vi "44xxRefClk.vi"(8 "error in (no error)":errorcluster, 9 "DAQ Type":T1, 10 "ActiveDev":tag, 11 "Refnum in":refnum<k21>) -> (0 "error out":errorcluster, 2 "RefClk.Src":tag, 3 "Refnum out":refnum<k21>)   [LabVIEW 2016, in "Instrument.Lockin.lvclass"]
uses:
  Instrument.Lockin.lvclass
  Typedefs/DAQType-enum.ctl
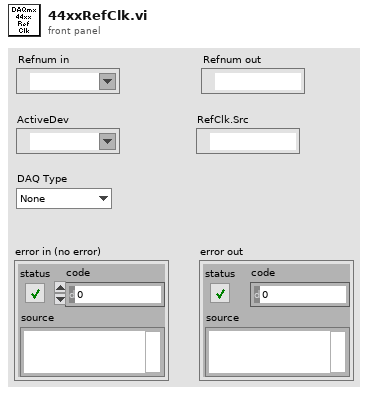
[diagram p1: front panel]
types:
  T1 = typedef "Instrument.Lockin.lvclass/DAQType-enum.ctl" = enum16{"None", "USB 4431", "PXI 446x"}
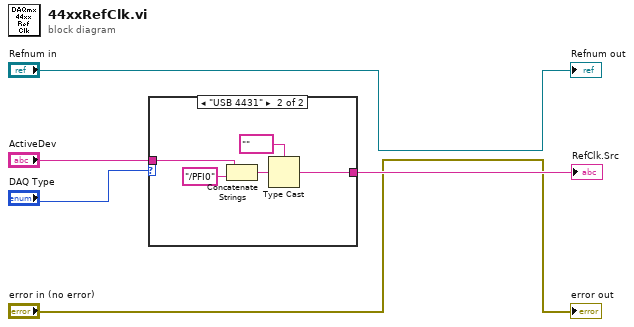
[diagram p0: block diagram]
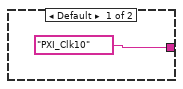
[diagram p2: hidden frame]
diagram:
  n1 = case shown="\"USB 4431\"" "DAQ Type" {
    tunnel: [tag "PXI_Clk10" ("RefClk.Src") w8] -> w3
    tunnel: "ActiveDev" -> [_ w7]
    frame Default {
    }
    frame "USB 4431" {
      n2 = Concatenate Strings(w7, "/PFI0" ("string")) -> (w9:string)
      n3 = Type Cast(type=tag "" ("RefClk.Src"), x=w9) -> (*(type *) &x=w8:tag)
    }
  }
  "RefClk.Src" <- w3
  "error out" <- "error in (no error)"
  "Refnum out" <- "Refnum in"
